vi "TryToConnect.vi"(8 "error in":errorcluster, 10 "timeout":i32=500, 11 "server in":refnum<class "RT FlexRIO Server TCP.lvclass">) -> (0 "error out":errorcluster, 3 "server out":refnum<class "RT FlexRIO Server TCP.lvclass">)   [LabVIEW 2017, in "RT FlexRIO Server TCP.lvclass"]
uses:
  RT FlexRIO Server TCP.lvclass
  Public/State.ctl
  Properties/TcpListener_GET.vi
  Properties/Connection_SET.vi
  Properties/State_SET.vi
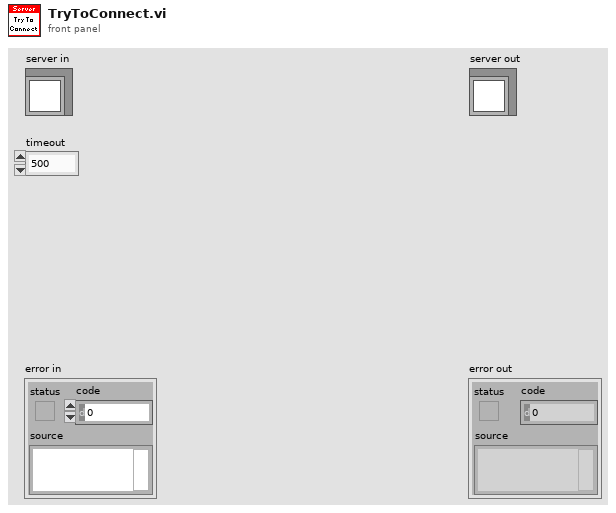
[diagram p1: front panel]
types:
  T1 = typedef "RT FlexRIO Server TCP.lvclass/State.ctl" = enum16{"started", "connected", "stopped"}
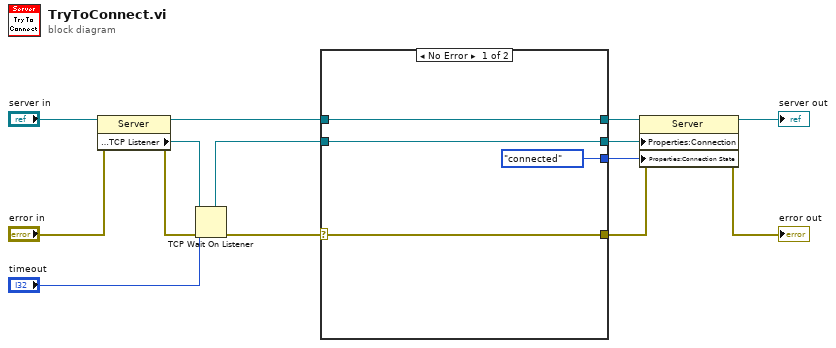
[diagram p0: block diagram]
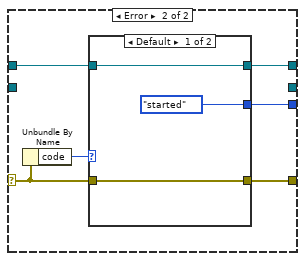
[diagram p2: hidden frame]
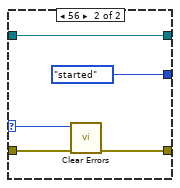
[diagram p3: hidden frame]
diagram:
  n1 = property class="Server"(reference="server in", error in="error in") -> (reference out=w8:refnum<class "RT FlexRIO Server TCP.lvclass">, error out=w11:errorcluster, "Properties:TCP Listener"=w9:refnum<k5>)
  n2 = TCP Wait On Listener(8:w11, 9:"timeout", 11:w9) -> (0:w10:errorcluster, 4:w7:refnum<k5>)  [unwired: 1 in, 3 out]
  n3 = case shown="No Error" w10 {
    selector: w10 -> [w16 w22]
    tunnel: [w16 w23] -> w5
    tunnel: w8 -> [w18 w19]
    tunnel: [w18 w20] -> w2
    tunnel: w7 -> [w17 _]
    tunnel: [w17 _] -> w3
    tunnel: [State."connected" ("connection state") w21] -> w1
    frame No Error {
    }
    frame Error {
      n4 = Unbundle By Name(w22) -> ("code"=w24:i32)
      n5 = case shown="Default" w24 {
        selector: w24 -> [_ w30]
        tunnel: [w27 w31] -> w23
        tunnel: w22 -> [w27 w32]
        tunnel: [State."started" ("connection state") State."started" ("connection state")] -> w21
        tunnel: [w25 w28] -> w20
        tunnel: w19 -> [w25 w28]
        frame Default {
        }
        frame 56 {
          n6 = call <vilib>:"Clear Errors.vi"("error in (no error)"=w32, "specific error code to clear (0: all)"=w30) -> ("error out"=w31:errorcluster)  [unwired: 4 in, 1 out]
        }
      }
    }
  }
  n7 = property class="Server"(reference=w2, error in=w5, "Properties:Connection"=w3, "Properties:Connection State"=w1) -> (reference out=→"server out":refnum<class "RT FlexRIO Server TCP.lvclass">, error out=→"error out":errorcluster)
